vi "GetPlayerInformation.vi"(8 "error in (no error)":errorcluster, 11 "ClashRoyale in":refnum<class "StashRoyale.lvclass">) -> (0 "error out":errorcluster, 3 "ClashRoyale out":refnum<class "StashRoyale.lvclass">)   [LabVIEW 2020, in "StashRoyale.lvclass"]
uses:
  StashRoyale.lvclass
  StashRoyale.lvclass/StashRoyale.ctl
  ctl_ClientError.ctl
  ctl_Player.ctl
  <vilib>/httpClient/LabVIEWHTTPClient.lvlib
  <vilib>/addons/Tools/Unicode/UTF8 Tools.lvlib
  support/JSON.lvlibp
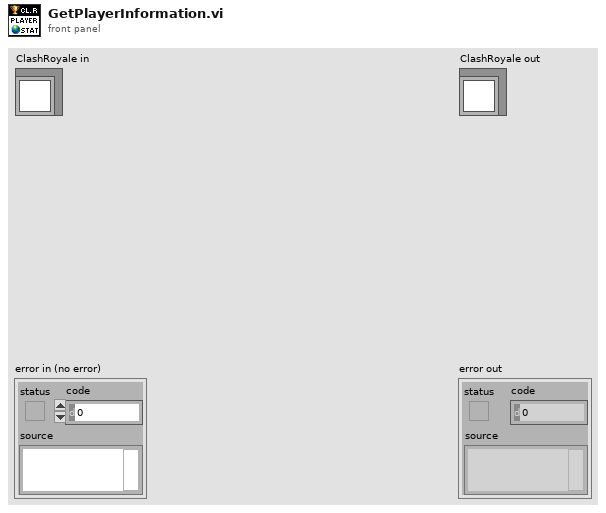
[diagram p1: front panel]
types:
  T1 = typedef "LabVIEWHTTPClient.lvlib/ClientHandle.ctl" = refnum<k1>
  T2 = typedef "StashRoyale.lvclass/ctl_ErrorCodes.ctl" = i32
  T3 = typedef "StashRoyale.lvclass/ctl_ClientError.ctl" = cluster{"reason":string, "message":string, "type":string}
  T4 = typedef "StashRoyale.lvclass/ctl_Player.ctl" = cluster{"name":string, "expLevel":u8, "trophies":u16, "bestTrophies":u16, "wins":u16, "losses":u16, "battleCount":u16, "threeCrownWins":u16}
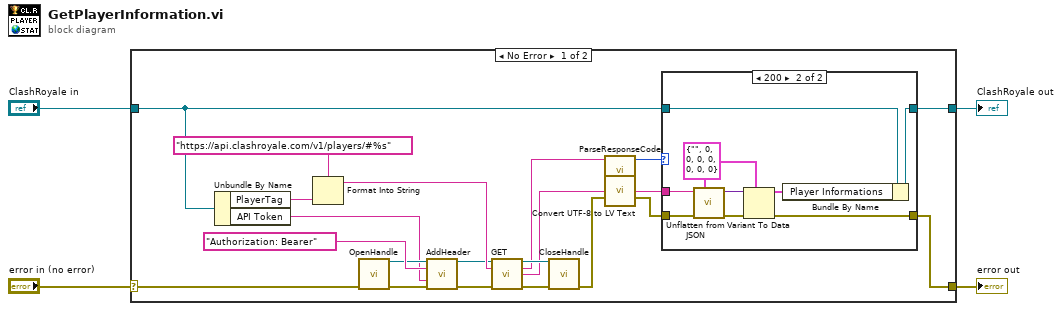
[diagram p0: block diagram]
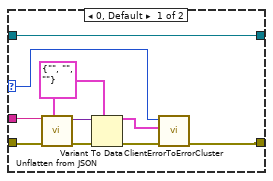
[diagram p2: hidden frame]
diagram:
  n1 = case shown="No Error" "error in (no error)" {
    selector: "error in (no error)" -> [w22 w46]
    tunnel: [w7 w46] -> w3
    tunnel: [w17 w45] -> w1
    tunnel: "ClashRoyale in" -> [w19 w45]
    frame No Error {
      n2 = Unbundle By Name(w19) -> ("PlayerTag"=w18:string, "API Token"=w10:string)
      n3 = Format Into String(format string="https://api.clashroyale.com/v1/players/#%s" ("url"), w18) -> (resulting string=w20:string)  [unwired: 2 in, 1 out]
      n4 = call <vilib>:"OpenHandle.vi"("error in (no error)"=w22) -> ("client handle out"=w14:T1, "error out"=w11:errorcluster)  [unwired: 13 in]
      n5 = call <vilib>:"AddHeader.vi"("client handle"=w14, "header"="Authorization: Bearer", "value"=w10, "error in (no error)"=w11) -> ("client handle out"=w13:T1, "error out"=w12:errorcluster)  [unwired: 10 in]
      n6 = call <vilib>:"GET.vi"("client handle"=w13, "url"=w20, "error in (no error)"=w12) -> ("client handle out"=w25:T1, "headers"=w6:string, "body"=w23:string, "error out"=w24:errorcluster)  [unwired: 9 in]
      n7 = call <vilib>:"CloseHandle.vi"("client handle"=w25, "error in (no error)"=w24) -> ("error out"=w16:errorcluster)  [unwired: 13 in]
      n8 = call "ParseResponseCode.vi"("Response Header"=w6) -> ("response code (200)"=w5:T2)  [unwired: 10 in]
      n9 = call <vilib>:"Convert UTF-8 to LV Text.vi"("UTF-8 Text"=w23, "error in"=w16) -> ("LV Text"=w9:string, "error out"=w8:errorcluster)  [unwired: 12 in]
      n10 = case shown="200" w5 {
        selector: w5 -> [w27 _]
        tunnel: w19 -> [w35 w44]
        tunnel: [w35 w43] -> w17
        tunnel: w9 -> [w32 w39]
        tunnel: w8 -> [w31 w37]
        tunnel: [w26 w36] -> w7
        frame 0, Default {
          w30 = T3 {"reason"="", "message"="", "type"=""} ("ClientError")
          n11 = call "Unflatten from JSON.vi"("Type and Defaults"=w30, "error in (no error)"=w31, "JSON String"=w32) -> ("error out"=w33:errorcluster, "data"=w34:variant)  [unwired: 7 in]
          n12 = Variant To Data(error in=w33, type=w30, Variant=w34) -> (data=w28:T3, error out=w29:errorcluster)
          n13 = call "ClientErrorToErrorCluster.vi"("error in (no error)"=w29, "ClientError"=w28, "response code (200)"=w27) -> ("error out"=w26:errorcluster)  [unwired: 8 in]
        }
        frame 200 {
          w41 = T4 {"name"="", "expLevel"=0, "trophies"=0, "bestTrophies"=0, "wins"=0, "losses"=0, "battleCount"=0, "threeCrownWins"=0} ("Player")
          n14 = call "Unflatten from JSON.vi"("Type and Defaults"=w41, "error in (no error)"=w37, "JSON String"=w39) -> ("error out"=w38:errorcluster, "data"=w42:variant)  [unwired: 7 in]
          n15 = Variant To Data(error in=w38, type=w41, Variant=w42) -> (data=w40:T4, error out=w36:errorcluster)
          n16 = Bundle By Name(cluster=w44, "Player Informations"=w40) -> (w43:refnum<class "StashRoyale.lvclass">)
        }
      }
    }
    frame Error {
    }
  }
  "error out" <- w3
  "ClashRoyale out" <- w1
